vi "Library_General_init.vi"(8 "error in (no error)":errorcluster) -> (0 "error out":errorcluster)   [LabVIEW 2013]
uses:
  My Computer/Controls/Sepios General Parameters.ctl
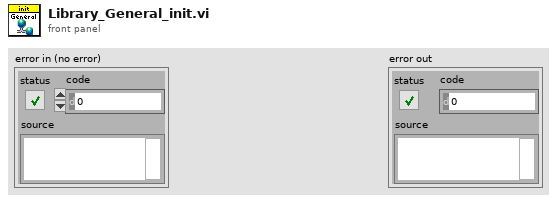
[diagram p1: front panel]
types:
  T1 = typedef "Sepios General Parameters.ctl" = cluster{"Sensors-Settings":cluster{"Water density [kg/m3]":dbl, "SB_parameters":cluster{"x0":dbl, "U_full":dbl, "U_empty":dbl}}, "Startup":cluster{"Enable Swimbladder":bool}, "Default Configuration File":path}
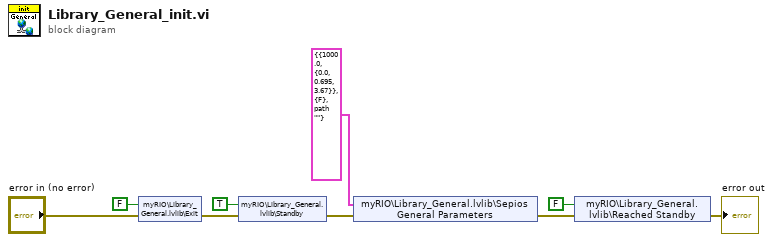
[diagram p0: block diagram]
diagram:
  n1 = shared-variable "myRIO\\Library_General.lvlib\\Exit"(FALSE ("Exit"), error in="error in (no error)") -> (error out=w5:errorcluster)
  n2 = shared-variable "myRIO\\Library_General.lvlib\\Standby"(TRUE ("Running"), error in=w5) -> (error out=w4:errorcluster)
  n3 = shared-variable "myRIO\\Library_General.lvlib\\Sepios General Parameters"(T1 {"Sensors-Settings"={"Water density [kg/m3]"=1000.0, "SB_parameters"={"x0"=0.0, "U_full"=0.695, "U_empty"=3.67}}, "Startup"={"Enable Swimbladder"=FALSE}, "Default Configuration File"=path ""} ("Sepios General Parameters"), error in=w4) -> (error out=w3:errorcluster)
  n4 = shared-variable "myRIO\\Library_General.lvlib\\Reached Standby"(FALSE ("Reached Standby"), error in=w3) -> (error out=→"error out":errorcluster)
